vi "Proto Parser.vi"(8 "error in (no error)":errorcluster, 11 ".proto file path":path=path "C:/dev/labview-grpc-server/tests/data_marshal/data_marshal.proto") -> (0 "error out":errorcluster, 1 "gRPC Method Parameters":T4[](array[typedef]), 2 "gRPC Messages Parameters":T1[](array[typedef]))   [LabVIEW 2020, in "gRPC Scripting Tools.lvlib"]
uses:
  gRPC Scripting Tools.lvlib
  TypeDefs/RPC Method Parameters.ctl
  TypeDefs/Message Metadata (Scripting).ctl
  TypeDefs/Message Element Metadata (Scripting).ctl
  TypeDefs/Message Element Type.ctl
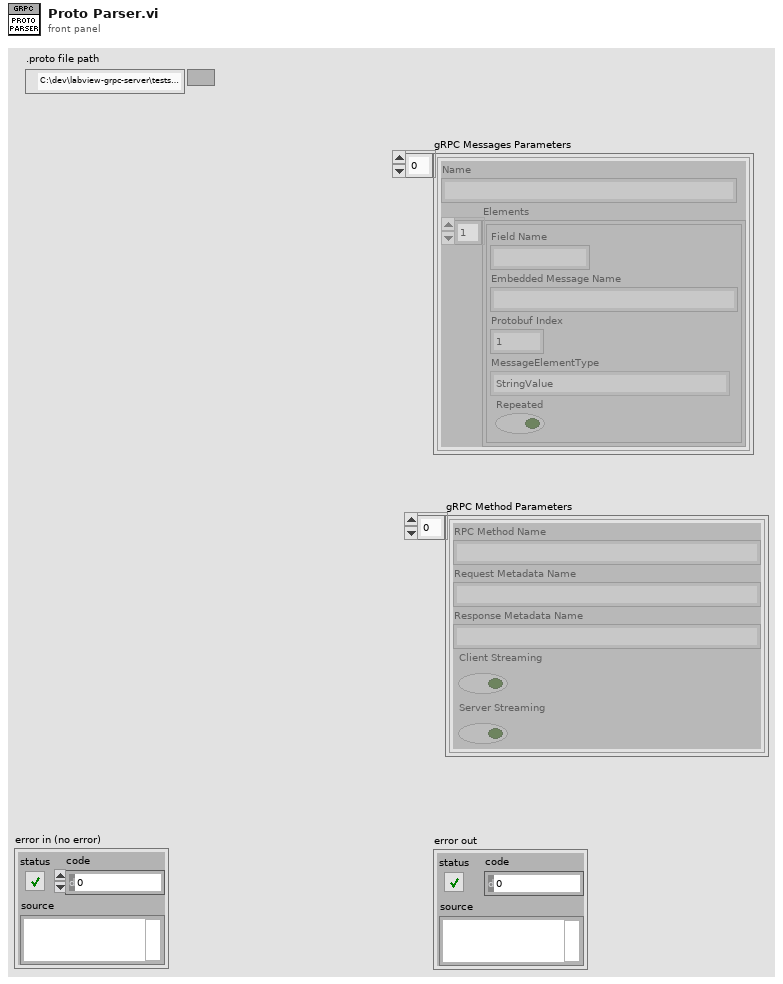
[diagram p1: front panel]
types:
  T1 = typedef "gRPC Scripting Tools.lvlib/Message Metadata (Scripting).ctl" = cluster{"Name":string, "Elements":T2[]}
  T2 = typedef "gRPC Scripting Tools.lvlib/Message Element Metadata (Scripting).ctl" = cluster{"Field Name":string, "Embedded Message Name":string, "Protobuf Index":i32, "MessageElementType":T3, "Repeated":bool}
  T3 = typedef "gRPC Scripting Tools.lvlib/Message Element Type.ctl" = enum32{"Int32Value", "FloatValue", "DoubleValue", "BoolValue", "StringValue", "MessageValue", "Int64Value", "UInt32Value", "UInt64Value", "EnumValue"}
  T4 = typedef "gRPC Scripting Tools.lvlib/RPC Method Parameters.ctl" = cluster{"RPC Method Name":string, "Request Metadata Name":string, "Response Metadata Name":string, "Client Streaming":bool, "Server Streaming":bool}
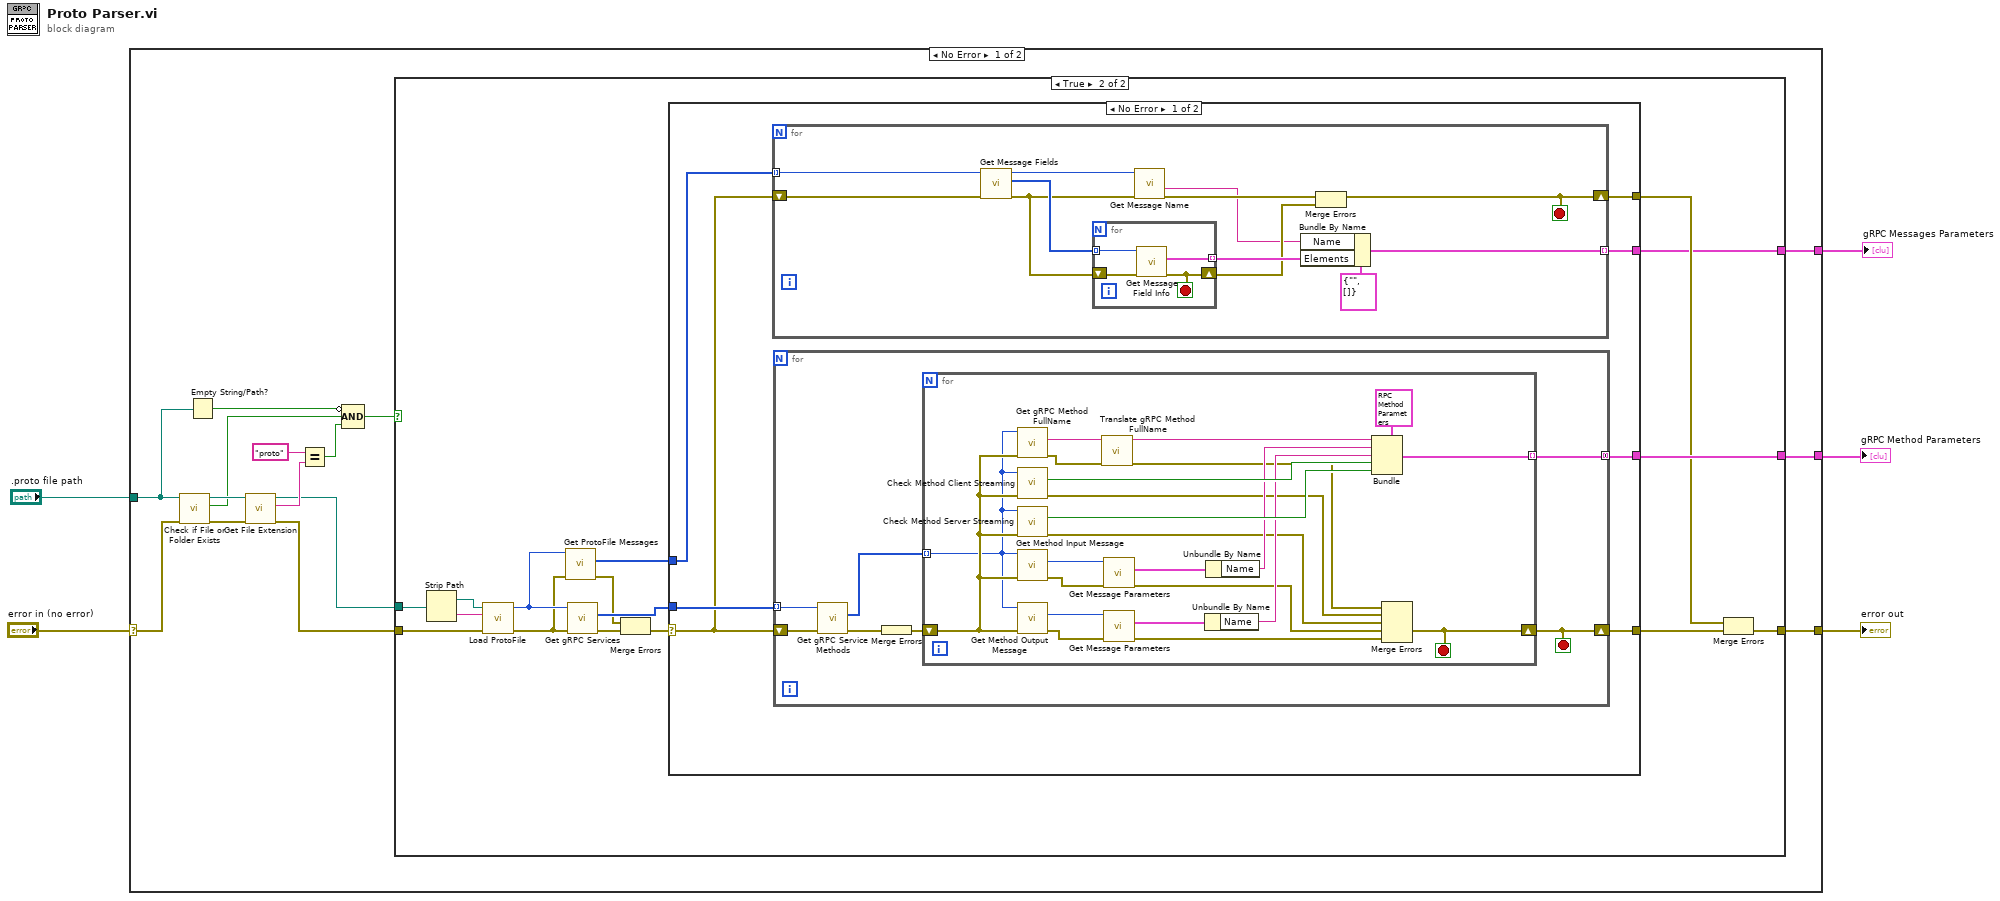
[diagram p0: block diagram]
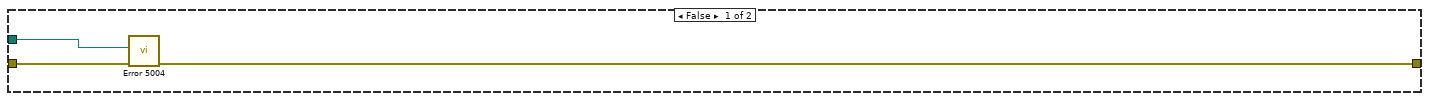
[diagram p2: hidden frame]
diagram:
  n1 = case shown="No Error" "error in (no error)" {
    selector: "error in (no error)" -> [w17 w94]
    tunnel: ".proto file path" -> [w18 _]
    tunnel: [w20 _] -> w5
    tunnel: [w19 w94] -> w4
    tunnel: [w6 _] -> w1
    frame No Error {
      n2 = call <vilib>:"Check if File or Folder Exists.vi"("error in (no error)"=w17, "path"=w18) -> ("error out"=w16:errorcluster, "file or folder exists?"=w11:bool, "dup path"=w15:path)  [unwired: 7 in]
      n3 = Empty String/Path?(string/path=w18) -> (empty?=w10:bool)
      n4 = call <vilib>:"Get File Extension.vi"("error in (no error)"=w16, "file"=w15) -> ("error out"=w7:errorcluster, "lowercase file extension"=w14:string, "dup file"=w8:path)  [unwired: 5 in, 2 out]
      n5 = Equal?(x="proto", y=w14) -> (x = y?=w12:bool)
      n6 = Compound Arithmetic op=AND(invert w10, w11, w12) -> (w9:bool)
      n7 = case shown="True" w9 {
        tunnel: [_ w36] -> w20
        tunnel: [w22 w25] -> w19
        tunnel: w8 -> [w21 w35]
        tunnel: w7 -> [w23 w34]
        tunnel: [_ w24] -> w6
        frame False {
          n8 = call "Error 5004.vi"("error in (no error)"=w23, "Proto file path"=w21) -> ("error out"=w22:errorcluster)  [unwired: 9 in]
        }
        frame True {
          n9 = Strip Path(path=w35) -> (stripped path=w39:path, name=w38:string)
          n10 = call "Load ProtoFile.vi"("error in (no error)"=w34, "File Name"=w38, "File Base path"=w39) -> ("error out"=w31:errorcluster, "protoFile ref out"=w32:u64)  [unwired: 7 in]
          n11 = call "Get ProtoFile Messages.vi"("error in (no error)"=w31, "Protofile ref in"=w32) -> ("error out"=w30:errorcluster, "ProtoFile Messages"=w28:u64[])  [unwired: 7 in, 1 out]
          n12 = call "Get gRPC Services.vi"("error in (no error)"=w31, "protoFile ref in"=w32) -> ("error out"=w33:errorcluster, "services"=w37:u64[])  [unwired: 7 in, 1 out]
          n13 = Merge Errors(w30, w33) -> (w29:errorcluster)
          n14 = case shown="No Error" w29 {
            selector: w29 -> [w42 w93]
            tunnel: w37 -> [w46 _]
            tunnel: [w45 _] -> w36
            tunnel: [w44 w93] -> w27
            tunnel: w28 -> [w43 _]
            tunnel: [w41 _] -> w26
            tunnel: [w40 _] -> w24
            frame No Error {
              n15 = for {
                tunnel: w43 -> [w58] mode=indexing
                shift-right: [w48] -> w41
                shift-left: w42 -> [w53]
                tunnel: [w49] -> w40 mode=indexing
                stop <- w48 stop-if-true
                n16 = call "Get Message Fields.vi"("error in (no error)"=w53, "Message ref in"=w58) -> ("error out"=w52:errorcluster, "Field refs"=w57:u64[], "Message ref out"=w56:u64)  [unwired: 7 in]
                n17 = for {
                  tunnel: w57 -> [w62] mode=indexing
                  tunnel: [w61] -> w54 mode=indexing
                  shift-right: [w59] -> w51
                  shift-left: w52 -> [w60]
                  stop <- w59 stop-if-true
                  n18 = call "Get Message Field Info.vi"("error in (no error)"=w60, "Message Field ref in"=w62) -> ("error out"=w59:errorcluster, "Field Info"=w61:T2)  [unwired: 7 in, 1 out]
                }
                n19 = call "Get Message Name.vi"("error in (no error)"=w52, "Message ref in"=w56) -> ("error out"=w50:errorcluster, "Message Name"=w47:string)  [unwired: 7 in, 1 out]
                n20 = Bundle By Name(cluster=T1 {"Name"="", "Elements"=[]} ("Message Metadata"), "Name"=w47, "Elements"=w54) -> (w49:T1)
                n21 = Merge Errors(w50, w51) -> (w48:errorcluster)
              }
              n22 = for {
                tunnel: w46 -> [w69] mode=indexing
                tunnel: [w68] -> w45 mode=concatenating
                shift-right: [w63] -> w44
                shift-left: w42 -> [w66]
                stop <- w63 stop-if-true
                n23 = call "Get gRPC Service Methods.vi"("error in (no error)"=w66, "Service ref in"=w69) -> ("error out"=w65:errorcluster, "Service Methods"=w67:u64[])  [unwired: 7 in, 1 out]
                n24 = Merge Errors(w65) -> (w64:errorcluster)
                n25 = for {
                  tunnel: w67 -> [w74] mode=indexing
                  tunnel: [w92] -> w68 mode=indexing
                  shift-right: [w76] -> w63
                  shift-left: w64 -> [w75]
                  stop <- w76 stop-if-true
                  n26 = call "Get gRPC Method FullName.vi"("error in (no error)"=w75, "Method ref in"=w74) -> ("error out"=w73:errorcluster, "Method Full Name"=w72:string)  [unwired: 7 in, 1 out]
                  n27 = call "Check Method Client Streaming.vi"("error in (no error)"=w75, "Method ref in"=w74) -> ("error out"=w80:errorcluster, "is Client Streaming"=w91:bool)  [unwired: 7 in, 1 out]
                  n28 = call "Check Method Server Streaming.vi"("error in (no error)"=w75, "Method ref in"=w74) -> ("error out"=w79:errorcluster, "is Server Streaming"=w90:bool)  [unwired: 7 in, 1 out]
                  n29 = call "Get Method Input Message.vi"("error in (no error)"=w75, "Method ref in"=w74) -> ("error out"=w85:errorcluster, "Message ref out"=w88:u64)  [unwired: 7 in, 1 out]
                  n30 = call "Get Method Output Message.vi"("error in (no error)"=w75, "Method ref in"=w74) -> ("error out"=w86:errorcluster, "Message ref out"=w87:u64)  [unwired: 7 in, 1 out]
                  n31 = call "Translate gRPC Method FullName.vi"("error in (no error)"=w73, "Method Full Name in"=w72) -> ("error out"=w70:errorcluster, "Method Full Name out"=w71:string)  [unwired: 8 in]
                  n32 = call "Get Message Parameters.vi"("error in (no error)"=w85, "Message ref in"=w88) -> ("error out"=w78:errorcluster, "Message Metadata"=w82:T1)  [unwired: 7 in, 1 out]
                  n33 = call "Get Message Parameters.vi"("error in (no error)"=w86, "Message ref in"=w87) -> ("error out"=w77:errorcluster, "Message Metadata"=w81:T1)  [unwired: 7 in, 1 out]
                  n34 = Unbundle By Name(w81) -> ("Name"=w83:string)
                  n35 = Unbundle By Name(w82) -> ("Name"=w84:string)
                  n36 = Bundle(cluster=T4 {"RPC Method Name"="/queryserver.QueryServer/Invoke", "Request Metadata Name"="InvokeRequest", "Response Metadata Name"="InvokeResponse", "Client Streaming"=FALSE, "Server Streaming"=FALSE}, "RPC Method Name"=w71, "Request Metadata Name"=w84, "Response Metadata Name"=w83, "Client Streaming"=w91, "Server Streaming"=w90) -> (w92:T4)
                  n37 = Merge Errors(w70, w80, w79, w78, w77) -> (w76:errorcluster)
                }
              }
            }
            frame Error {
            }
          }
          n38 = Merge Errors(w26, w27) -> (w25:errorcluster)
        }
      }
    }
    frame Error {
    }
  }
  "gRPC Method Parameters" <- w5
  "error out" <- w4
  "gRPC Messages Parameters" <- w1
